vi "init_sCMOS.vi"(0 "sCMOS_1":bool) -> (1 "Binning":dbl, 2 "Exposure":dbl, 3 "sCMOS init":cluster{"init":i16, "sCMOS handle":u32})   [LabVIEW 2015]
panel:
  in  "sCMOS":cluster{"init":i16, "sCMOS handle":u32}
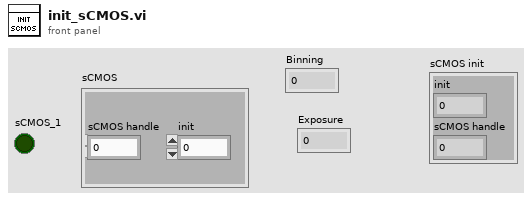
[diagram p1: front panel]
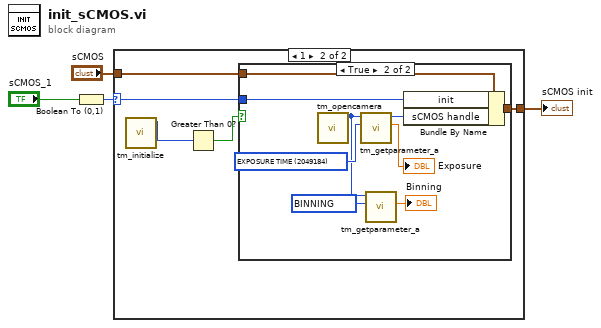
[diagram p0: block diagram]
diagram:
  n1 = Boolean To (0,1)(Boolean="sCMOS_1") -> (0, 1=w3:i16)
  n2 = case shown="1" w3 {
    selector: w3 -> [_ w9]
    tunnel: "sCMOS" -> [w5 w10]
    tunnel: [w5 w8] -> w1
    frame 0, Default {
    }
    frame 1 {
      n3 = call <userlib>:"tm_initialize.vi"() -> ("Number Of Cameras"=w7:u32)  [unwired: 8 in, 3 out]
      n4 = Greater Than 0?(x=w7) -> (x > 0?=w6:bool)
      n5 = case shown="True" w6 {
        tunnel: w10 -> [w11 w20]
        tunnel: w9 -> [_ w19]
        tunnel: [w11 w17] -> w8
        frame False {
        }
        frame True {
          w13 = u32 4215968 items=["SENSOR MODE"=4212128, "CCD MODE"=4212384, "READOUT MODE"=4211872, "ACTIVE VIEW INDEX"=4343136, "BITS PER CHANNEL"=4342976, "IMAGE PIXEL TYPE"=4343296, "BINNING"=4215968, "EXPOSURE TIME"=2049184, "CONTRAST GAIN"=3163312, "CONTRAST OFFSET"=3163328, "LIGHT MODE"=2114720, "SENSITIVITY"=2114992, "PHOTON IMAGING MODE"=2115200, "HIGH DYNAMIC RANGE MODE"=3163360, "WHITE BALANCE"=3163568, "TEMPERATURE"=2115232, "TEMPERATURE TARGET"=2115264, "SENSOR COOLER FAN"=2115296, "LINEBUNDLE HEIGHT"=4212192, "MECHANICAL SHUTTER"=2115488, "BACK FOCUS POSITION"=8422304, "TRIGGER CONNECTOR"=1066432, "TRIGGER SOURCE"=1066144, "OUTPUT TRIGGER SOURCE"=1852576, "TRIGGER GLOBAL EXPOSURE"=2049680, "FIRST TRIGGER BEHAVIOR"=2049696, "CHANNEL SYNC"=1852352, "READOUT DIRECTION"=4211904, "PRE HSYNC COUNT"=1852704, "INTERNAL LINE SPEED"=4226000, "INTERNAL LINE INTERVAL"=4226016] ("Parameter")
          w16 = u32 2049184 items=["SENSOR MODE"=4212128, "CCD MODE"=4212384, "READOUT MODE"=4211872, "ACTIVE VIEW INDEX"=4343136, "BITS PER CHANNEL"=4342976, "IMAGE PIXEL TYPE"=4343296, "BINNING"=4215968, "EXPOSURE TIME"=2049184, "CONTRAST GAIN"=3163312, "CONTRAST OFFSET"=3163328, "LIGHT MODE"=2114720, "SENSITIVITY"=2114992, "PHOTON IMAGING MODE"=2115200, "HIGH DYNAMIC RANGE MODE"=3163360, "WHITE BALANCE"=3163568, "TEMPERATURE"=2115232, "TEMPERATURE TARGET"=2115264, "SENSOR COOLER FAN"=2115296, "LINEBUNDLE HEIGHT"=4212192, "MECHANICAL SHUTTER"=2115488, "BACK FOCUS POSITION"=8422304, "TRIGGER CONNECTOR"=1066432, "TRIGGER SOURCE"=1066144, "OUTPUT TRIGGER SOURCE"=1852576, "TRIGGER GLOBAL EXPOSURE"=2049680, "FIRST TRIGGER BEHAVIOR"=2049696, "CHANNEL SYNC"=1852352, "READOUT DIRECTION"=4211904, "PRE HSYNC COUNT"=1852704, "INTERNAL LINE SPEED"=4226000, "INTERNAL LINE INTERVAL"=4226016] ("Parameter")
          n6 = call <userlib>:"tm_opencamera.vi"() -> ("Handle out"=w14:u32)  [unwired: 9 in, 2 out]
          n7 = call <userlib>:"tm_getparameter_a.vi"("Parameter"=w16, "Handle in"=w14) -> ("Value out"=→"Exposure":dbl, "Handle out"=w15:u32)  [unwired: 7 in, 1 out]
          n8 = call <userlib>:"tm_getparameter_a.vi"("Parameter"=w13, "Handle in"=w14) -> ("Value out"=→"Binning":dbl)  [unwired: 7 in, 2 out]
          n9 = Bundle By Name(cluster=w20, "init"=w19, "sCMOS handle"=w15) -> (w17:cluster{"init":i16, "sCMOS handle":u32})
        }
      }
    }
  }
  "sCMOS init" <- w1
